vi "VisionDistanceFromAngle.vi"(9 "Ty":dbl, 10 "Camera Height[in.]":dbl=30.0, 11 "Target Height[in.]":dbl=100.0) -> (3 "Dist. From Target[in.]":dbl)   [LabVIEW 2019]
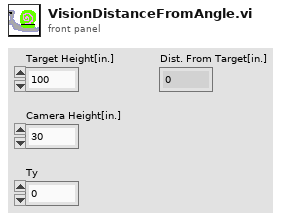
[diagram p1: front panel]
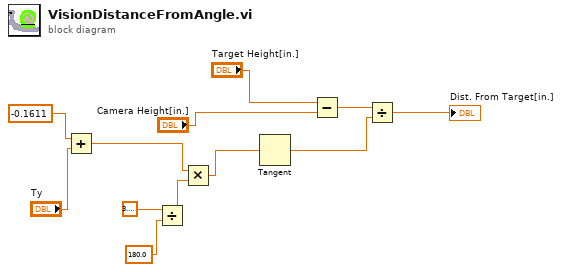
[diagram p0: block diagram]
diagram:
  n1 = Add(x=-0.1611, y="Ty") -> (x+y=w3:dbl)
  n2 = Divide(x=3.141592653589793, y=180.0) -> (x/y=w4:dbl)
  n3 = Multiply(x=w3, y=w4) -> (x*y=w7:dbl)
  n4 = Tangent(1:w7) -> (0:w8:dbl)
  n5 = Subtract(x="Target Height[in.]", y="Camera Height[in.]") -> (x-y=w9:dbl)
  n6 = Divide(x=w9, y=w8) -> (x/y=→"Dist. From Target[in.]":dbl)
